vi "item select tree calc.vi"(9 "indices":i32[](array[numeric]), 11 "selection states":bool[](array[boolean])) -> (3 "symbol state":T1)   [LabVIEW 2020, in "UI_ItemSelect.lvlib"]
uses:
  UI_ItemSelect.lvlib
  checkbox state.ctl
  <userlib>/_OpenG.lib/array/array.llb/Index 1D Array Elements (Boolean)__ogtk.vi
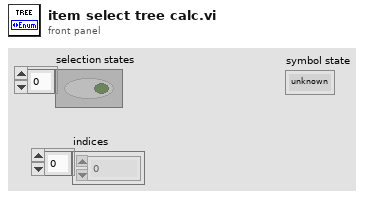
[diagram p1: front panel]
types:
  T1 = typedef "UI_ItemSelect.lvlib/checkbox state.ctl" = enum16{"unknown", "check", "some", "no check"}
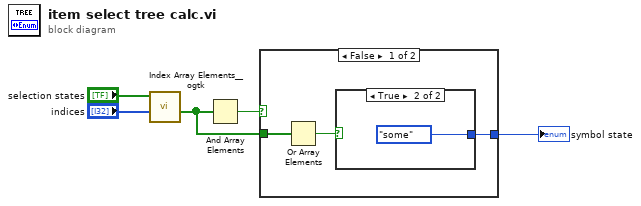
[diagram p0: block diagram]
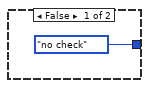
[diagram p2: hidden frame]
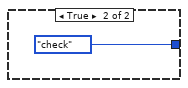
[diagram p3: hidden frame]
diagram:
  n1 = call-poly <userlib>:"Index Array Elements__ogtk.vi"("indices"="indices", "array"="selection states") -> ("elements"=w4:bool[])  [unwired: 9 in]
  n2 = And Array Elements(Boolean array=w4) -> (logical AND=w5:bool)
  n3 = case shown="False" w5 {
    tunnel: w4 -> [w8 _]
    tunnel: [w6 checkbox_state."check"] -> w1
    frame False {
      n4 = Or Array Elements(Boolean array=w8) -> (logical OR=w7:bool)
      n5 = case shown="True" w7 {
        tunnel: [checkbox_state."no check" checkbox_state."some"] -> w6
        frame False {
        }
        frame True {
        }
      }
    }
    frame True {
    }
  }
  "symbol state" <- w1
